vi "logging_set.vi"(8 "error in":errorcluster caption="error in (no error)", 10 "Logging target":string, 11 "VISA resource name":refnum<visa-resource-name>) -> (0 "error out":errorcluster, 3 "VISA resource name out":refnum<visa-resource-name>)   [LabVIEW 2020, in "Rohde&Schwarz RTx Oscilloscopes.lvlib" / "rsidr_core.lvlib"]
uses:
  rsidr_core.lvlib
  _type_Logging_Parameter.ctl
  type_Error_Codes.ctl
  Match Regular Expression.xnode
panel:
  # "Supported formats:\nUDP:<Local_Port>:<Remote_Port>:<Remote_Host>\n         e.g. UDP:61556:61557:localhost -alias=\nFILE:0-new/1-add:<path>"
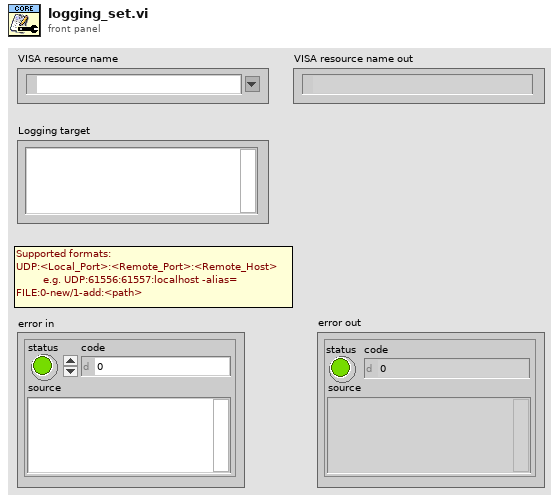
[diagram p1: front panel]
types:
  T1 = typedef "Rohde&Schwarz RTx Oscilloscopes.lvlib/rsidr_core.lvlib/_type_Logging_Parameter.ctl" = enum16{"Type (String)", "SessionAlias(String)", "FormatString (String)", "UDPconectionID (I32)", "UDPlocalPort (I32)", "UDPremotePort (I32)", "UDPremoteHost (String)", "FILEmode (I32)", "FILEpath (String)", "FILEopenID (I32)", "DataMaxLogLen (I32)"}
  T2 = enum16{"open", "replace", "create", "open or create", "replace or create", "replace or create with confirmation"}
  T3 = typedef "Rohde&Schwarz RTx Oscilloscopes.lvlib/rsidr_core.lvlib/type_Error_Codes.ctl" = enum16{"No_error", "VISA_err_ResourceNotFound", "VISA_err_Timeout", "VISA_warn_MoreDataAvailable", "RS_err_MissingCallback", "RS_err_InvalidAttribute", "RS_err_InvalidValue", "RS_err_UnknownResource", "RS_err_AlreadyInitialized", "RS_err_InstrumentStatus", "RS_err_BadRepCapName", "RS_err_TypesMismatch", "RS_err_ValueNotSupported", "RS_err_InvalidRngTable", "RS_err_IDqueryFail", "RS_err_UnexpResponse", "VISA_warn_ConfigNotLoaded", "RS_err_AttributeNotReadable", "RS_err_AttributeNotWritable", "RS_err_InstrumentType", "RS_err_InstrumentOption", "VISA_err_InvalidSize", "RS_err_ReliabilityIndicator", "VISA_warn_UnknownStatus", "VISA_warn_TermCharRead", "VISA_err_IO_error", "RS_err_FunctionNotSupported", "VISA_warn_QueueEmpty"}
  T4 = typedef "Rohde&Schwarz RTx Oscilloscopes.lvlib/rsidr_core.lvlib/type_Session_Data.ctl" = cluster{"IDN string":string, "Instrument FW":string, "Instr type":string, "Instr type for err. msg.":string, "Installed Options":string[], "Ignore Error Messages":string, "Logging params":variant, "OPC Timeout":i32, "VISA Timeout":i32, "STB Poll VISA Timeout":i32, "Additional Flags":i32, "Wait Before Read":i32, "Wait Before Write":i32, "Option String Flags":i32, "IO Segment Size":i64, "VISA Access Mode":T5, "Interface Type":T6, "OPC Wait Mode":T7, "Bin Float Number  Format":T8, "Bin Integer Number Format":T9, "Simulate":bool, "VXIcapable":bool, "Duplicate Session":bool, "Add LF to Write":bool, "Logging":bool, "Fast Sweep":bool, "Query Instrument Status":bool, "Check Range":bool, "Check Options":bool, "OPC-sync Attr Writes":bool, "OPC-sync Attr Queries":bool}
  T5 = typedef "Rohde&Schwarz RTx Oscilloscopes.lvlib/rsidr_core.lvlib/type_VisaAccessMode.ctl" = u16
  T6 = typedef "Rohde&Schwarz RTx Oscilloscopes.lvlib/rsidr_core.lvlib/type_InterfaceType.ctl" = enum16{"Unknown", "GPIB", "VXI", "GPIB_VXI", "ASRL", "PXI", "TCPIP", "USB", "SOCKET"}
  T7 = typedef "Rohde&Schwarz RTx Oscilloscopes.lvlib/rsidr_core.lvlib/type_OPC_Wait_Mode.ctl" = enum16{"STBpolling", "STBpollingSlow", "STBpollingSuperSlow", "ServiceRequest", "OPCquery"}
  T8 = typedef "Rohde&Schwarz RTx Oscilloscopes.lvlib/rsidr_core.lvlib/type_Binary_Float_Number_Format.ctl" = enum16{"Float_4_Bytes_Swapped", "Float_4_Bytes", "Double_8_Bytes_Swapped", "Double_8_Bytes"}
  T9 = typedef "Rohde&Schwarz RTx Oscilloscopes.lvlib/rsidr_core.lvlib/type_Binary_Integer_Number_Format.ctl" = enum16{"Int32_4_Bytes_Swapped", "Int32_4 Bytes", "Int16_2_Bytes_Swapped", "Int16_2_Bytes"}
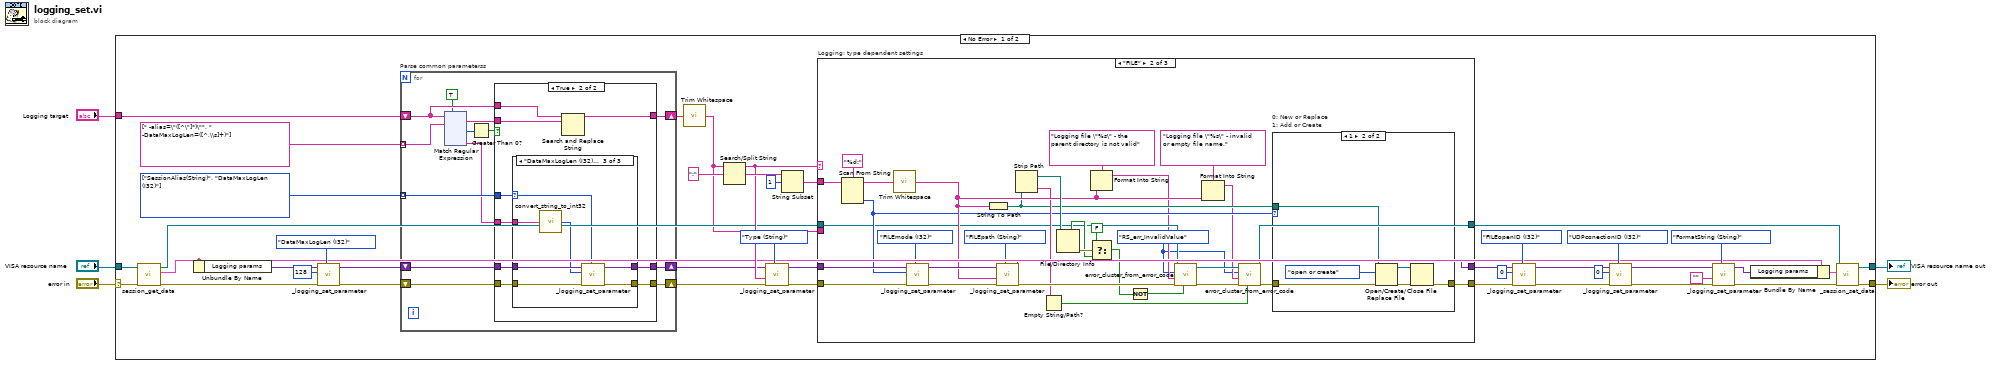
[diagram p0: block diagram]
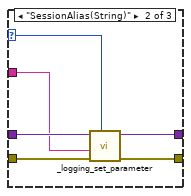
[diagram p4: hidden frame]
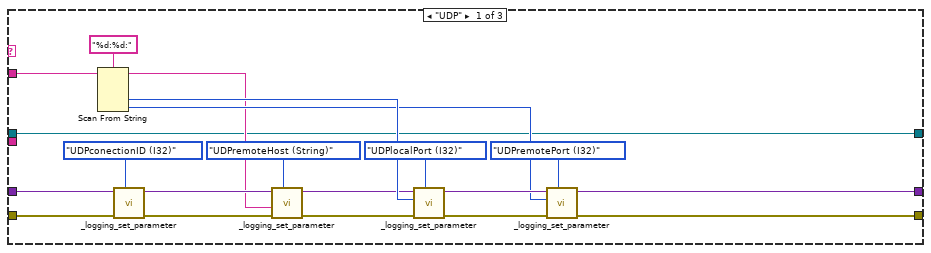
[diagram p5: hidden frame]
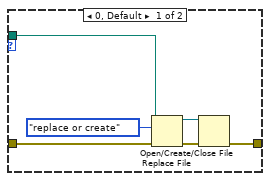
[diagram p6: hidden frame]
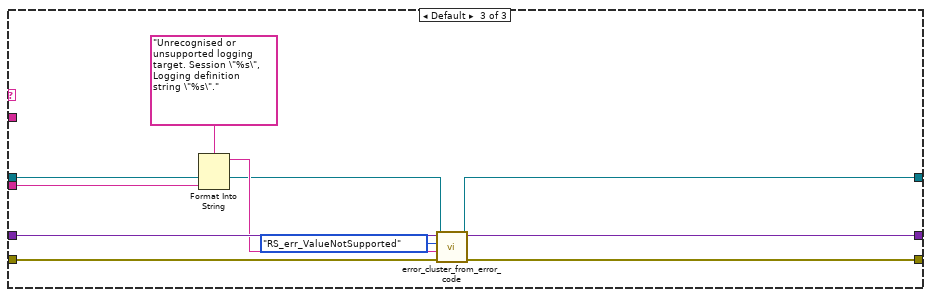
[diagram p7: hidden frame]
diagram:
  n1 = case shown="No Error" "error in" {
    selector: "error in" -> [w44 w277]
    tunnel: [w43 w277] -> w2
    tunnel: "VISA resource name" -> [w19 w276]
    tunnel: "Logging target" -> [w23 _]
    tunnel: [w42 w276] -> w1
    frame No Error {
      w17 = T1[] [enum."SessionAlias(String)", enum."DataMaxLogLen (I32)"] items=["Type (String)", "SessionAlias(String)", "FormatString (String)", "UDPconectionID (I32)", "UDPlocalPort (I32)", "UDPremotePort (I32)", "UDPremoteHost (String)", "FILEmode (I32)", "FILEpath (String)", "FILEopenID (I32)", "DataMaxLogLen (I32)"]
      n2 = call "session_get_data.vi"("error in"=w44, "VISA resource name"=w19) -> ("error out"=w10:errorcluster, "Session User Data out"=w8:T4, "VISA resource name out"=w32:refnum<visa-resource-name>)  [unwired: 6 in, 1 out]
      n3 = Unbundle By Name(w8) -> ("Logging params"=w9:variant)
      n4 = call "_logging_set_parameter.vi"("Logging Parameter"=_type_Logging_Parameter."DataMaxLogLen (I32)", "error in"=w10, "Int32 parameter (0)"=128 ("I32 parameter (0)"), "Logging params in"=w9) -> ("error out"=w6:errorcluster, "Logging params out"=w7:variant)  [unwired: 6 in]
      n5 = for "Parse common parameterss" {
        shift-right: [w58] -> w21
        shift-left: w23 -> [w59]
        tunnel: string[] [" -alias=\"([^\"]*)\"", " -DataMaxLogLen=([^,\\s]+)"] -> [w61] mode=indexing
        shift-right: [w54] -> w18
        shift-left: w7 -> [w57]
        tunnel: w17 -> [w56] mode=indexing
        shift-right: [w53] -> w16
        shift-left: w6 -> [w55]
        n6 = xnode ("Match Regular Expression")("input string"=w59, "regular expression"=w61, "ignore case? (F)"=TRUE) -> ("whole match"=w60:string, "offset past match"=w52:i32, "submatch 1"=w49:string)  [unwired: 3 in, 3 out]
        n7 = Greater Than 0?(x=w52) -> (x > 0?=w51:bool)
        n8 = case shown="True" w51 {
          tunnel: w60 -> [_ w71]
          tunnel: w59 -> [w64 w72]
          tunnel: [w64 w73] -> w58
          tunnel: w57 -> [w63 w68]
          tunnel: w49 -> [_ w66]
          tunnel: w56 -> [_ w69]
          tunnel: w55 -> [w62 w70]
          tunnel: [w63 w67] -> w54
          tunnel: [w62 w65] -> w53
          frame False {
          }
          frame True {
            n9 = case shown="\"DataMaxLogLen (I32)\"" w69 {
              selector: w69 -> [_ w78 w85]
              tunnel: w70 -> [w74 w81 w88]
              tunnel: w68 -> [w75 w80 w87]
              tunnel: [w75 w79 w86] -> w67
              tunnel: w66 -> [_ w77 w83]
              tunnel: [w74 w76 w84] -> w65
              frame Default {
              }
              frame "SessionAlias(String)" {
                n10 = call "_logging_set_parameter.vi"("Logging Parameter"=w78, "error in"=w81, "String parameter (\"\")"=w77, "Logging params in"=w80) -> ("error out"=w76:errorcluster, "Logging params out"=w79:variant)  [unwired: 6 in]
              }
              frame "DataMaxLogLen (I32)" {
                n11 = call "convert_string_to_int32.vi"("String in"=w83) -> ("int32 value out"=w82:i32)  [unwired: 4 in]
                n12 = call "_logging_set_parameter.vi"("Logging Parameter"=w85, "error in"=w88, "Int32 parameter (0)"=w82, "Logging params in"=w87) -> ("error out"=w84:errorcluster, "Logging params out"=w86:variant)  [unwired: 6 in]
              }
            }
            n13 = Search and Replace String(input string=w72, search string=w71) -> (result string=w73:string)  [unwired: 6 in, 3 out]
          }
        }
      }
      n14 = call "Trim Whitespace.vi"("string"=w21) -> ("trimmed string"=w20:string)  [unwired: 1 in]
      n15 = Search/Split String(string=w20, search string/char (-)=":") -> (substring before match=w38:string, match + rest of string=w47:string)  [unwired: 1 in, 1 out]
      n16 = call "_logging_set_parameter.vi"("Logging Parameter"=_type_Logging_Parameter."Type (String)", "error in"=w16, "String parameter (\"\")"=w38, "Logging params in"=w18) -> ("error out"=w40:errorcluster, "Logging params out"=w39:variant)  [unwired: 6 in]
      n17 = String Subset(string=w47, offset (0)=1) -> (substring=w45:string)  [unwired: 1 in]
      n18 = case "Logging: type dependent settings" shown="\"FILE\"" w38 {
        tunnel: w40 -> [w220 w250 w272]
        tunnel: w45 -> [w221 w254 _]
        tunnel: w39 -> [w205 w251 w271]
        tunnel: [w219 w228 w275] -> w27
        tunnel: w20 -> [_ _ w274]
        tunnel: w32 -> [w202 w227 w268]
        tunnel: [w204 w232 w271] -> w25
        tunnel: [w202 w225 w267] -> w15
        frame "UDP" {
          n19 = Scan From String(format string="%d:%d:", input string=w221) -> (remaining string=w203:string, output 1=w212:i32, output 2=w206:i32)  [unwired: 4 in, 2 out]
          n20 = call "_logging_set_parameter.vi"("Logging Parameter"=_type_Logging_Parameter."UDPconectionID (I32)", "error in"=w220, "Logging params in"=w205) -> ("error out"=w215:errorcluster, "Logging params out"=w214:variant)  [unwired: 7 in]
          n21 = call "_logging_set_parameter.vi"("Logging Parameter"=_type_Logging_Parameter."UDPremoteHost (String)", "error in"=w215, "String parameter (\"\")"=w203, "Logging params in"=w214) -> ("error out"=w210:errorcluster, "Logging params out"=w207:variant)  [unwired: 6 in]
          n22 = call "_logging_set_parameter.vi"("Logging Parameter"=_type_Logging_Parameter."UDPlocalPort (I32)", "error in"=w210, "Int32 parameter (0)"=w212, "Logging params in"=w207) -> ("error out"=w209:errorcluster, "Logging params out"=w208:variant)  [unwired: 6 in]
          n23 = call "_logging_set_parameter.vi"("Logging Parameter"=_type_Logging_Parameter."UDPremotePort (I32)", "error in"=w209, "Int32 parameter (0)"=w206, "Logging params in"=w208) -> ("error out"=w219:errorcluster, "Logging params out"=w204:variant)  [unwired: 6 in]
        }
        frame "FILE" {
          w222 = type_Error_Codes."RS_err_InvalidValue" ("Error Enum in")
          n24 = Scan From String(format string="%d:", input string=w254) -> (remaining string=w236:string, output 1=w231:i32)  [unwired: 3 in, 2 out]
          n25 = call "Trim Whitespace.vi"("string"=w236) -> ("trimmed string"=w235:string)  [unwired: 1 in]
          n26 = call "_logging_set_parameter.vi"("Logging Parameter"=_type_Logging_Parameter."FILEmode (I32)", "error in"=w250, "Int32 parameter (0)"=w231, "Logging params in"=w251) -> ("error out"=w249:errorcluster, "Logging params out"=w247:variant)  [unwired: 6 in]
          n27 = String To Path(string=w235) -> (path=w229:path)
          n28 = call "_logging_set_parameter.vi"("Logging Parameter"=_type_Logging_Parameter."FILEpath (String)", "error in"=w249, "String parameter (\"\")"=w235, "Logging params in"=w247) -> ("error out"=w246:errorcluster, "Logging params out"=w232:variant)  [unwired: 6 in]
          n29 = Strip Path(path=w229) -> (stripped path=w237:path, name=w233:string)
          n30 = Empty String/Path?(string/path=w233) -> (empty?=w234:bool)
          n31 = File/Directory Info(path=w237) -> (directory=w244:bool, error out=w245:errorcluster)  [unwired: 1 in, 5 out]
          n32 = Format Into String(format string="Logging file \"%s\" - the parent directory is not valid", w235) -> (resulting string=w223:string)  [unwired: 2 in, 1 out]
          n33 = Select(t=FALSE, s=w245, f=w244) -> (s? t:f=w242:bool)
          n34 = Not(x=w242) -> (.not. x?=w241:bool)
          n35 = call "error_cluster_from_error_code.vi"("Error Creation Enabled (True)"=w241, "error in"=w246, "Error Message (\"\")"=w223, "Error Enum in"=w222, "VISA resource name"=w227) -> ("error out"=w239:errorcluster, "VISA resource name out"=w226:refnum<visa-resource-name>)  [unwired: 5 in]
          n36 = Format Into String(format string="Logging file \"%s\" - invalid or empty file name.", w235) -> (resulting string=w224:string)  [unwired: 2 in, 1 out]
          n37 = call "error_cluster_from_error_code.vi"("Error Creation Enabled (True)"=w234, "error in"=w239, "Error Message (\"\")"=w224, "Error Enum in"=w222, "VISA resource name"=w226) -> ("error out"=w230:errorcluster, "VISA resource name out"=w225:refnum<visa-resource-name>)  [unwired: 5 in]
          n38 = case "0: New or Replace\n1: Add or Create" shown="1" w231 {
            tunnel: w230 -> [w260 w266]
            tunnel: w229 -> [w259 w265]
            tunnel: [w255 w261] -> w228
            frame 0, Default {
              n39 = Open/Create/Replace File(file path (use dialog)=w259, error in=w260, operation (0:open)=T2."replace or create") -> (refnum out=w256:refnum<file>, error out=w257:errorcluster)  [unwired: 3 in, 1 out]
              n40 = Close File(refnum=w256, error in=w257) -> (error out=w255:errorcluster)  [unwired: 1 out]
            }
            frame 1 {
              n41 = Open/Create/Replace File(file path (use dialog)=w265, error in=w266, operation (0:open)=T2."open or create") -> (refnum out=w262:refnum<file>, error out=w263:errorcluster)  [unwired: 3 in, 1 out]
              n42 = Close File(refnum=w262, error in=w263) -> (error out=w261:errorcluster)  [unwired: 1 out]
            }
          }
        }
        frame Default {
          n43 = Format Into String(format string="Unrecognised or unsupported logging target. Session \"%s\", Logging definition string \"%s\".", w268, w274) -> (resulting string=w270:string)  [unwired: 2 in, 1 out]
          n44 = call "error_cluster_from_error_code.vi"("error in"=w272, "Error Message (\"\")"=w270, "Error Enum in"=type_Error_Codes."RS_err_ValueNotSupported", "VISA resource name"=w268) -> ("error out"=w275:errorcluster, "VISA resource name out"=w267:refnum<visa-resource-name>)  [unwired: 6 in]
        }
      }
      n45 = call "_logging_set_parameter.vi"("Logging Parameter"=_type_Logging_Parameter."FILEopenID (I32)", "error in"=w27, "Int32 parameter (0)"=0 ("I32 parameter (0)"), "Logging params in"=w25) -> ("error out"=w26:errorcluster, "Logging params out"=w24:variant)  [unwired: 6 in]
      n46 = call "_logging_set_parameter.vi"("Logging Parameter"=_type_Logging_Parameter."UDPconectionID (I32)", "error in"=w26, "Int32 parameter (0)"=0 ("I32 parameter (0)"), "Logging params in"=w24) -> ("error out"=w35:errorcluster, "Logging params out"=w34:variant)  [unwired: 6 in]
      n47 = call "_logging_set_parameter.vi"("Logging Parameter"=_type_Logging_Parameter."FormatString (String)", "error in"=w35, "String parameter (\"\")"="" ("Empty String Constant"), "Logging params in"=w34) -> ("error out"=w13:errorcluster, "Logging params out"=w14:variant)  [unwired: 6 in]
      n48 = Bundle By Name(cluster=w8, "Logging params"=w14) -> (w33:T4)
      n49 = call "_session_set_data.vi"("error in"=w13, "Session User Data in"=w33, "VISA resource name"=w15) -> ("error out"=w43:errorcluster, "VISA resource name out"=w42:refnum<visa-resource-name>)  [unwired: 7 in]
    }
    frame Error {
    }
  }
  "VISA resource name out" <- w1
  "error out" <- w2
